vi "ReadExitEvent.vi"(8 "ErrorIn":errorcluster caption="Error In", 11 "YActorIn":refnum<class "YActor.lvclass"> caption="Object In") -> (0 "ErrorOut":errorcluster caption="Error Out", 2 "ExitEvent":refnum<user-event>, 3 "YActorOut":refnum<class "YActor.lvclass"> caption="Object Out")   [LabVIEW 2021, in "YActor.lvclass"]
uses:
  YActor.lvclass
  YActor.lvclass/YActor.ctl
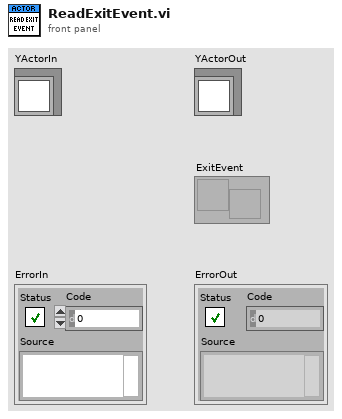
[diagram p1: front panel]
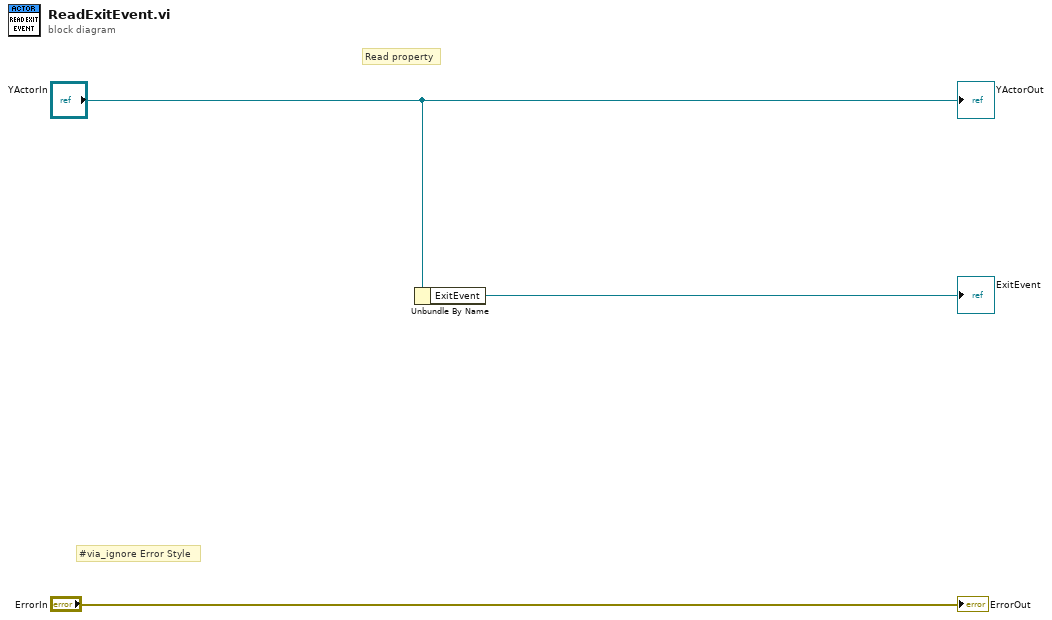
[diagram p0: block diagram]
diagram:
  # "#via_ignore Error Style"
  # "Read property"
  n1 = Unbundle By Name("YActorIn") -> ("ExitEvent"=→"ExitEvent":refnum<user-event>)
  "ErrorOut" <- "ErrorIn"
  "YActorOut" <- "YActorIn"
